vi "Configure.vi"(8 "error in (no error)":errorcluster, 11 "DC in":refnum<class "DC.lvclass">) -> (0 "error out":errorcluster, 3 "DC out":refnum<class "DC.lvclass">)   [LabVIEW 2020, in "DC.lvclass"]
doc: "Configure the measurements paramaters to sweep.\nThis should be a pop up interface invoked by the configure test button on the main panel."
uses:
  DC.lvclass
panel:
  in  "OK Button":bool
  in  "User Note":string
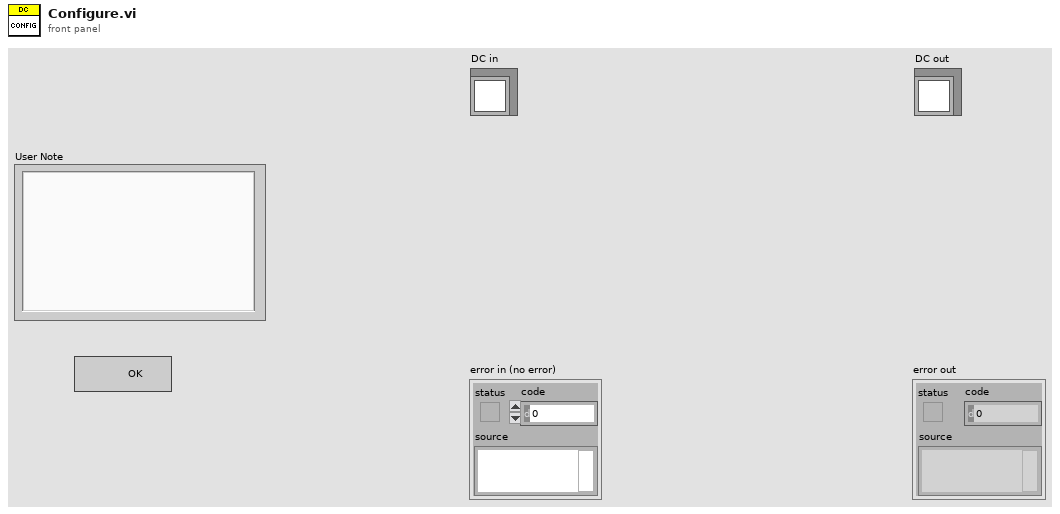
[diagram p1: front panel]
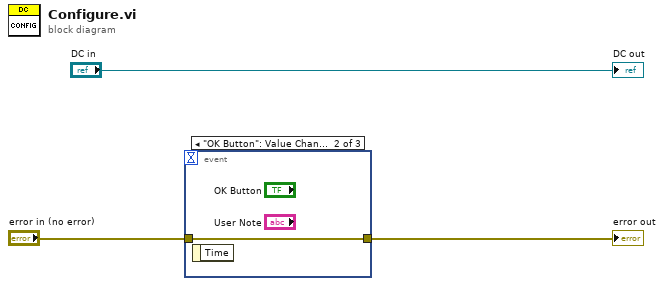
[diagram p0: block diagram]
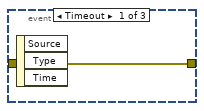
[diagram p2: hidden frame]
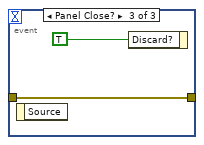
[diagram p3: hidden frame]
diagram:
  n1 = event shown="[1] \"OK Button\": Value Change" {
    selector: _ -> [_ _ _]
    dyn-events: _ -> [_ _ _]
    timeout: _ -> [_ _ _]
    tunnel: "error in (no error)" -> [w4 w5 w6]
    tunnel: [w4 w5 w6] -> w2
    event Timeout {
      n2 = event-data() -> ()  [unwired: 1 in, 3 out]
    }
    event "OK Button": Value Change {
      n3 = event-data() -> ()  [unwired: 1 in, 1 out]
    }
    event Panel Close? {
      n4 = event-data() -> ()  [unwired: 1 in, 1 out]
      n5 = event-data("Discard?"=TRUE) -> ()  [unwired: 1 in, 1 out]
    }
  }
  "error out" <- w2
  "DC out" <- "DC in"
